vi "Validate Credentials Domain.vi"(7 "domain":string, 8 "error in (no error)":errorcluster, 10 "password":string, 11 "userName":string) -> (0 "error out":errorcluster, 3 "valid":bool)   [LabVIEW 2017, in "Windows Security.lvlib"]
doc: "Validate the credentials against the domain."
uses:
  Windows Security.lvlib
  System.DirectoryServices.AccountManagement
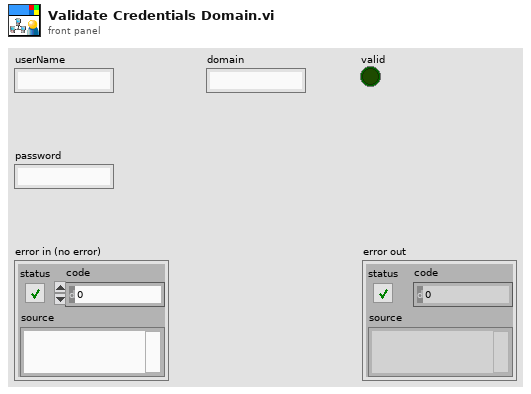
[diagram p1: front panel]
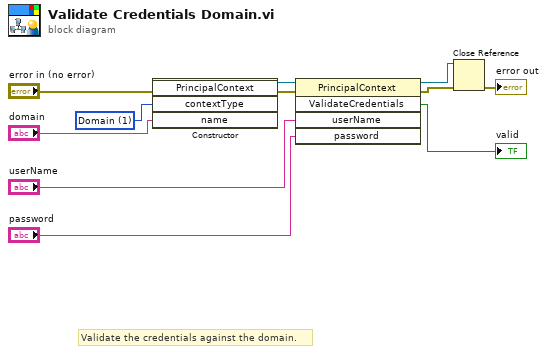
[diagram p0: block diagram]
diagram:
  w11 = 1 items=["Machine", "Domain", "ApplicationDirectory"] ("contextType")
  # "Validate the credentials against the domain."
  n1 = constructor class="PrincipalContext"(error in="error in (no error)", "contextType"=w11, "name"="domain") -> (reference out=w3:refnum<k24>, error out=w9:errorcluster)  [unwired: 2 in, 3 out]
  n2 = invoke class="PrincipalContext" method="ValidateCredentials"(reference=w3, error in=w9, "userName"="userName", "password"="password") -> (reference out=w1:refnum<k24>, error out=w8:errorcluster, "ValidateCredentials"=→"valid":bool)  [unwired: 1 in, 2 out]
  n3 = Close Reference(reference=w1, error in (no error)=w8) -> (error out=→"error out":errorcluster)
